vi "ss_walk_through_flywheel_sim.vi"(7 "init FlyWheelSim":T1 {"GearBox"."Jr_KgM2" format="%13.5p"; "GearBox"."L_H" format="%13.5p"; "GearBox"."Kt_NMPerAmp" format="%13.5p"; "GearBox"."KvINV_RadPerSecPerVolt" format="%13.5p"; "GearBox"."R_Ohms" format="%13.5p"; "GearBox"."FreeSpeed_RadPerSec" format="%13.5p"; "GearBox"."FreeCurrent_Amps" format="%13.5p"; "GearBox"."StallCurrent_Amps" format="%13.5p"; "GearBox"."StallTorque_NM" format="%13.5p"; "GearBox"."nominalVoltage_Volts" format="%13.5p"}, 8 "Cycle Time\nSeconds":dbl=0.02 format="%#_13g", 11 "Motor Dmd\nCO":dbl) -> (1 "Current Amps":dbl format="%20.3f", 2 "Battery Voltage":dbl, 3 "Speed Rad/Sec\nPV":dbl, 4 "out FlyWheelSim":T1 {"GearBox"."Jr_KgM2" format="%13.5p"; "GearBox"."L_H" format="%13.5p"; "GearBox"."Kt_NMPerAmp" format="%13.5p"; "GearBox"."KvINV_RadPerSecPerVolt" format="%13.5p"; "GearBox"."R_Ohms" format="%13.5p"; "GearBox"."FreeSpeed_RadPerSec" format="%13.5p"; "GearBox"."FreeCurrent_Amps" format="%13.5p"; "GearBox"."StallCurrent_Amps" format="%13.5p"; "GearBox"."StallTorque_NM" format="%13.5p"; "GearBox"."nominalVoltage_Volts" format="%13.5p"})   [LabVIEW 2019]
uses:
  <vilib>/Rock Robotics/WPI/ThirdParty/JAS_Junk/TrajLib/TypeDef/FLYWHEEL_SIM.ctl
  <vilib>/Rock Robotics/WPI/ThirdParty/JAS_Junk/TrajLib/TypeDef/LINEAR_SYSTEM_SIM.ctl
  <vilib>/Rock Robotics/WPI/ThirdParty/JAS_Junk/TrajLib/TypeDef/LINEAR_SYSTEM.ctl
  <vilib>/Analysis/Matrix/Datatypes/RealMatrix.ctl
  <vilib>/Rock Robotics/WPI/ThirdParty/JAS_Junk/TrajLib/TypeDef/DCMOTOR.CTL
  <vilib>/Rock Robotics/WPI/ThirdParty/JAS_Junk/TrajLib/Trajectory_Library.lvlib
  <vilib>/ptbypt/NI_PtbyPt.lvlib
  <vilib>/Analysis/Matrix/NI_Matrix.lvlib
panel:
  # "<States, 1>"
  # "<Outputs, 1>"
  # "<Inputs, 1>"
  # "<Outputs, 1>"
  # "<States,States>"
  # "<States,Inputs>"
  # "<Outputs,States>"
  # "<Outputs,Inputs>"
  # "<States, 1>"
  # "<Outputs, 1>"
  # "<Inputs, 1>"
  # "<Outputs, 1>"
  # "<States,States>"
  # "<States,Inputs>"
  # "<Outputs,States>"
  # "<Outputs,Inputs>"
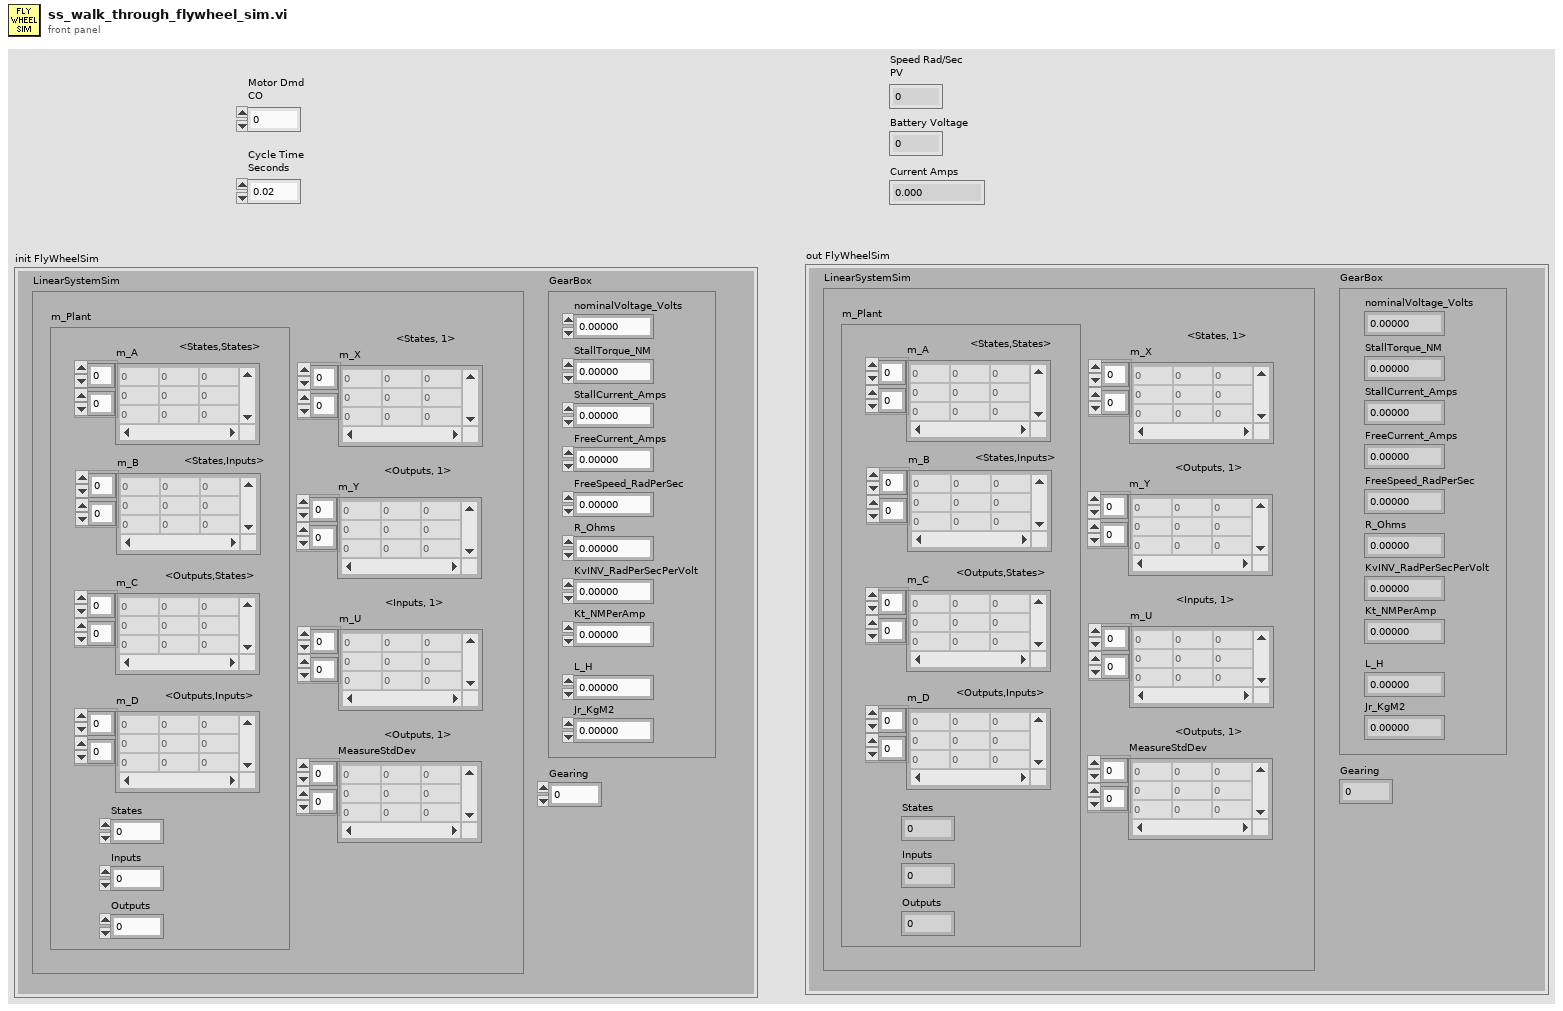
[diagram p1: front panel]
types:
  T1 = typedef "Trajectory_Library.lvlib/FLYWHEEL_SIM.ctl" = cluster{"LinearSystemSim":T2, "GearBox":T5, "Gearing":dbl}
  T2 = typedef "Trajectory_Library.lvlib/LINEAR_SYSTEM_SIM.ctl" = cluster{"m_Plant":T3, "m_X":T4, "m_Y":T4, "m_U":T4, "MeasureStdDev":T4}
  T3 = typedef "Trajectory_Library.lvlib/LINEAR_SYSTEM.ctl" = cluster{"m_A":T4, "m_B":T4, "m_C":T4, "m_D":T4, "States":i32, "Inputs":i32, "Outputs":i32}
  T4 = typedef "NI_Matrix.lvlib/RealMatrix.ctl" = dbl[][]
  T5 = typedef "Trajectory_Library.lvlib/DCMOTOR.CTL" = cluster{"nominalVoltage_Volts":dbl, "StallTorque_NM":dbl, "StallCurrent_Amps":dbl, "FreeCurrent_Amps":dbl, "FreeSpeed_RadPerSec":dbl, "R_Ohms":dbl, "KvINV_RadPerSecPerVolt":dbl, "Kt_NMPerAmp":dbl, "L_H":dbl, "Jr_KgM2":dbl}
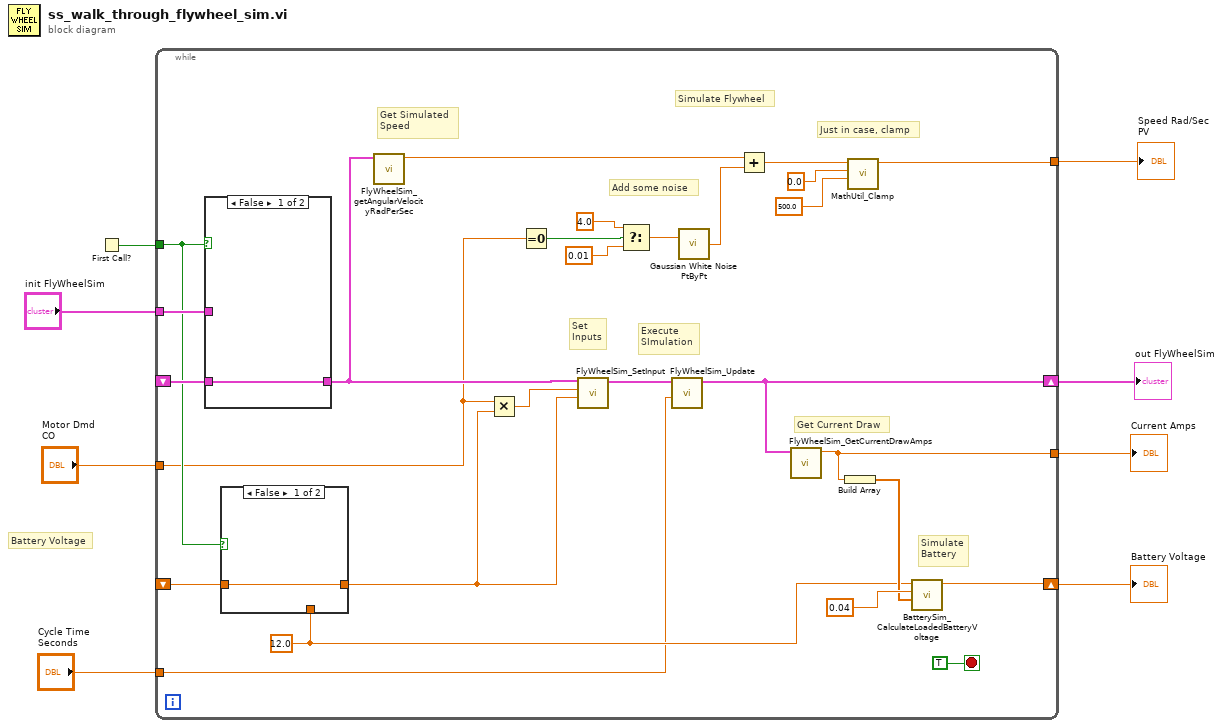
[diagram p0: block diagram]
diagram:
  # "Battery Voltage"
  n1 = First Call?() -> (First Call?: T/F=w7:bool)
  n2 = while {
    shift-right: [w31] -> w1
    shift-left: _ -> [w18]
    shift-right: [w28] -> w2
    shift-left: _ -> [w16]
    tunnel: "init FlyWheelSim" -> [w19]
    tunnel: w7 -> [w17]
    tunnel: "Motor Dmd\nCO" -> [w10]
    tunnel: [w13] -> w5
    tunnel: [w12] -> w4
    tunnel: "Cycle Time\nSeconds" -> [w9]
    stop <- TRUE stop-if-true
    w14 = 12.0
    # "Simulate\nBattery"
    # "Get Current Draw"
    # "Execute\nSImulation"
    # "Set\nInputs"
    # "Just in case, clamp"
    # "Get Simulated \nSpeed"
    # "Simulate Flywheel"
    # "Add some noise"
    n3 = case shown="False" w17 {
      tunnel: [w38 w39] -> w20
      tunnel: w19 -> [_ w39]
      tunnel: w18 -> [w38 _]
      frame False {
      }
      frame True {
      }
    }
    n4 = case shown="False" w17 {
      tunnel: w16 -> [w36 _]
      tunnel: [w36 w37] -> w15
      tunnel: w14 -> [_ w37]
      frame False {
      }
      frame True {
      }
    }
    n5 = call <vilib>:"FlyWheelSim_getAngularVelocityRadPerSec.vi"("FlyWheelSim"=w20) -> ("Velocity_RadPerSec"=w32:dbl)  [unwired: 10 in]
    n6 = Multiply(x=w10, y=w15) -> (x*y=w21:dbl)
    n7 = Equal To 0?(x=w10) -> (x = 0?=w11:bool)
    n8 = call <vilib>:"FlyWheelSim_SetInput.vi"("Battery_Volts"=w15, "Volts"=w21, "FlyWheelSim"=w20) -> ("out FlyWheelSim"=w33:T1)  [unwired: 8 in]
    n9 = Select(t=4.0 ("upper bound (100)"), s=w11, f=0.01) -> (s? t:f=w24:dbl)
    n10 = call <vilib>:"FlyWheelSim_Update.vi"("dT_Seconds"=w9, "FlyWheelSim"=w33) -> ("out FlyWheelSim"=w31:T1)  [unwired: 8 in, 1 out]
    n11 = call <vilib>:"Gaussian White Noise PtByPt.vi"("standard deviation"=w24) -> ("Gaussian white noise"=w34:dbl)  [unwired: 2 in]
    n12 = Add(x=w32, y=w34) -> (x+y=w25:dbl)
    n13 = call <vilib>:"FlyWheelSim_GetCurrentDrawAmps.vi"("FlyWheelSim"=w31) -> ("Current_Amps"=w13:dbl)  [unwired: 10 in]
    n14 = Build Array(w13) -> (w29:dbl[])
    n15 = call <vilib>:"MathUtil_Clamp.vi"("High Limit"=500.0, "Low Limit"=0.0, "Value"=w25) -> ("Result"=w12:dbl)  [unwired: 8 in]
    n16 = call <vilib>:"BatterySim_CalculateLoadedBatteryVoltage.vi"("Currents"=w29, "Resistance_Ohms"=0.04, "NominalVoltage"=w14) -> ("Voltage"=w28:dbl)  [unwired: 8 in]
  }
  "Current Amps" <- w5
  "Speed Rad/Sec\nPV" <- w4
  "Battery Voltage" <- w2
  "out FlyWheelSim" <- w1
